vi "Init.vi"(10 "Filename_Config":string) -> (0 "error out":errorcluster, 1 "VarsCount":i32, 2 "VarTree":T1 {"Rawdata" format="0x%08x"}, 3 "Init?":bool)   [LabVIEW 2014]
uses:
  _init_vartree/typedefs/ExVarTreeArray.ctl
  _init_vartree/typedefs/ExVarTree.ctl
  _init_vartree/typedefs/val_type_t.ctl
  type_def/DataCluster.ctl
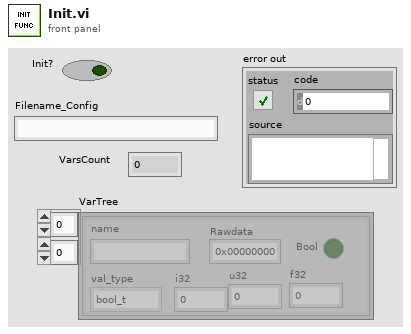
[diagram p1: front panel]
types:
  T1 = typedef "ExVarTreeArray.ctl" = T2[][]
  T2 = typedef "ExVarTree.ctl" = cluster{"name":string, "val_type":T3, "Rawdata":u32, "i32":i32, "u32":u32, "f32":sgl, "Bool":bool}
  T3 = typedef "val_type_t.ctl" = enum16{"bool_t", "i32_t", "u32_t", "f32_t"}
  T4 = typedef "DataCluster.ctl" = cluster{"Time":timestamp, "CommOK?":bool}
  T5 = typedef "vartree_t.ctl" = cluster{"names":string[], "vars":T6[], "ser_idxs":i32[], "perms":u8[]}
  T6 = typedef "var_t.ctl" = cluster{"data":u32, "val_type":T3}
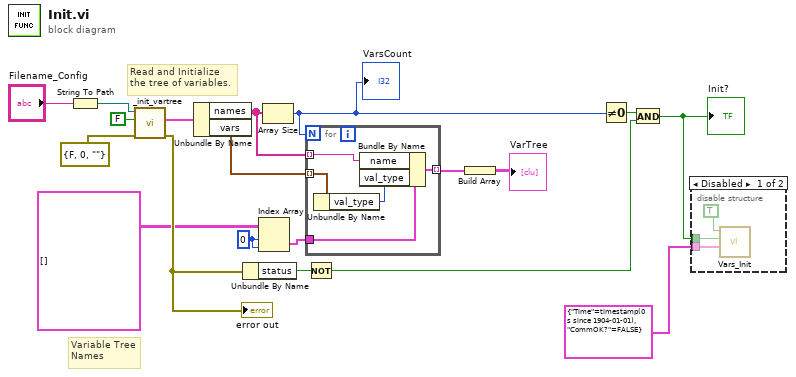
[diagram p0: block diagram]
diagram:
  w3 = 0 ("index (row)")
  # "Variable Tree\nNames"
  # "Read and Initialize \nthe tree of variables."
  n1 = String To Path(string="Filename_Config") -> (path=w11:path)
  n2 = call "_init_vartree.vi"("error in (no error)"=errorcluster {"status"=FALSE, "code"=0, "source"=""}, "config?"=FALSE, "appended path"=w11) -> ("error out"=w10:errorcluster, "vartree"=w19:T5)  [unwired: 7 in]
  "error out" <- w10
  n3 = Unbundle By Name(w19) -> ("names"=w9:string[], "vars"=w8:T6[])
  n4 = Unbundle By Name(w10) -> ("status"=w16:bool)
  n5 = Index Array(array=T1 [] ("VarTree"), index (row)=w3, index (col)=w3) -> (element=w7:T2)
  n6 = Array Size(array=w9) -> (size(s)=w4:i32)
  "VarsCount" <- w4
  n7 = for {
    N: w4 -> [_]
    tunnel: w9 -> [w23] mode=indexing
    tunnel: w8 -> [w22] mode=indexing
    tunnel: w7 -> [w24]
    tunnel: [w20] -> w2 mode=indexing
    n8 = Unbundle By Name(w22) -> ("val_type"=w21:T3)
    n9 = Bundle By Name(cluster=w24, "name"=w23, "val_type"=w21) -> (w20:T2)
  }
  n10 = Not(x=w16) -> (.not. x?=w17:bool)
  n11 = Build Array(w2) -> (→"VarTree":T2[][])
  n12 = Not Equal To 0?(x=w4) -> (x != 0?=w15:bool)
  n13 = And(x=w15, y=w17) -> (x .and. y?=w13:bool)
  "Init?" <- w13
  n14 = disable-structure shown="Disabled" {
    disable-tunnel: w13 -> [w26 _]
    disable-tunnel: T4 {"Time"=timestamp(0 s since 1904-01-01), "CommOK?"=FALSE} ("Cluster") -> [w25 _]
    frame Disabled {
      n15 = call "Vars_Init.vi"("Data Cluster In"=w25, "Init? In"=w26, "WriteVars?"=TRUE) -> ()  [unwired: 7 in, 2 out]
    }
    frame Enabled {
    }
  }
